vi "3.1.vi"() -> ()   [LabVIEW 2017]
panel:
  out "Numeric":dbl
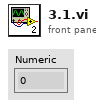
[diagram p1: front panel]
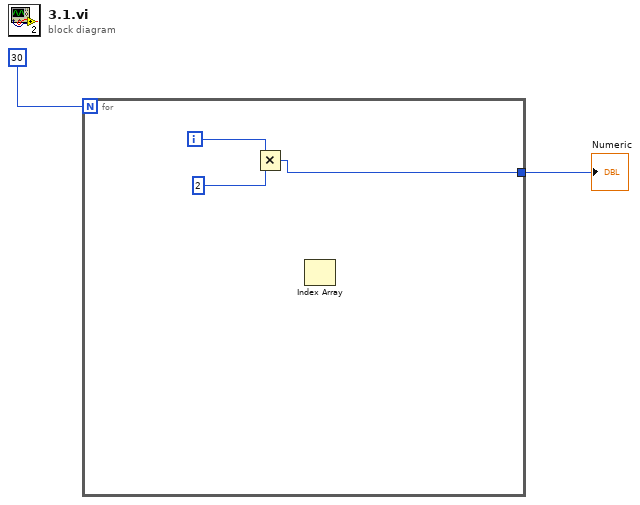
[diagram p0: block diagram]
diagram:
  n1 = for {
    N: 30 -> [_]
    tunnel: [w3] -> w1
    i -> [w4]
    n2 = Multiply(x=w4, y=2) -> (x*y=w3:i32)
    n3 = Index Array() -> ()  [unwired: 2 in, 1 out]
  }
  "Numeric" <- w1
